vi "Simulador 22_03.vi"() -> ()   [LabVIEW 2014]
uses:
  <vilib>/imath/engines/lvmath2/RunTimeEngine/Managers/WorkSpace/UID Generator.vi
  <vilib>/imath/engines/lvmath2/RunTimeEngine/RunTimeType/NIMS_RunTimeType_From StrictType (excl LVString).vi
  <instcachedir>/0/NIMS_RunTimeType_From StrictType (excl LVString)_15A5391EEA9C4AACB9955AC755B83D29.lvgen/NIMS_RunTimeType_From StrictType (excl LVString)_15A5391EEA9C4AACB9955AC755B83D29_000.vi
  <vilib>/imath/engines/lvmath2/RunTimeEngine/LocalVariableDefStatement/MC_LocalVariableDefStatement_Display.vi
  <vilib>/imath/engines/lvmath2/RunTimeEngine/ArithmeticOperatorToken/NIMS_ArithmeticOperator_power(S).vi
  <instcachedir>/0/NIMS_ArithmeticOperator_power(S)_CAFE680B12A64A3A8F5E28A20C679B7D.lvgen/NIMS_ArithmeticOperator_power(S)_CAFE680B12A64A3A8F5E28A20C679B7D_010.vi
  <vilib>/imathl/engines/lvmath/Functions/Error Handling/Create Error.vi
  <vilib>/imath/engines/lvmath2/RunTimeEngine/Managers/SymbolTable/Clear UID.vi
  <vilib>/imath/engines/lvmath2/RunTimeEngine/NodeEndStatement/NIMS_NodeEndStatement_Output.vi
  <instcachedir>/0/NIMS_NodeEndStatement_Output_53EC0D466D134D7ABD903AC30B43404B.lvgen/NIMS_NodeEndStatement_Output_53EC0D466D134D7ABD903AC30B43404B_010.vi
  <instcachedir>/0/NIMS_NodeEndStatement_Output_53EC0D466D134D7ABD903AC30B43404B.lvgen/NIMS_NodeEndStatement_Output_53EC0D466D134D7ABD903AC30B43404B_001.vi
  <vilib>/imath/engines/lvmath2/RunTimeEngine/ErrorHandling/NIMS_Finalize Error.vi
  <vilib>/imath/engines/lvmath2/RunTimeEngine/Managers/SymbolTable/NIMS_WorkSpace.lvlib
panel:
  in  "h":cdb
  in  "milliseconds to wait":u32
  out "y":dbl
  in  "Present (s)":dbl
  out "Waveform Chart":dbl(graph)
  in  "stop":bool
  out "Tank":dbl(slide) scale=0.0..30.0
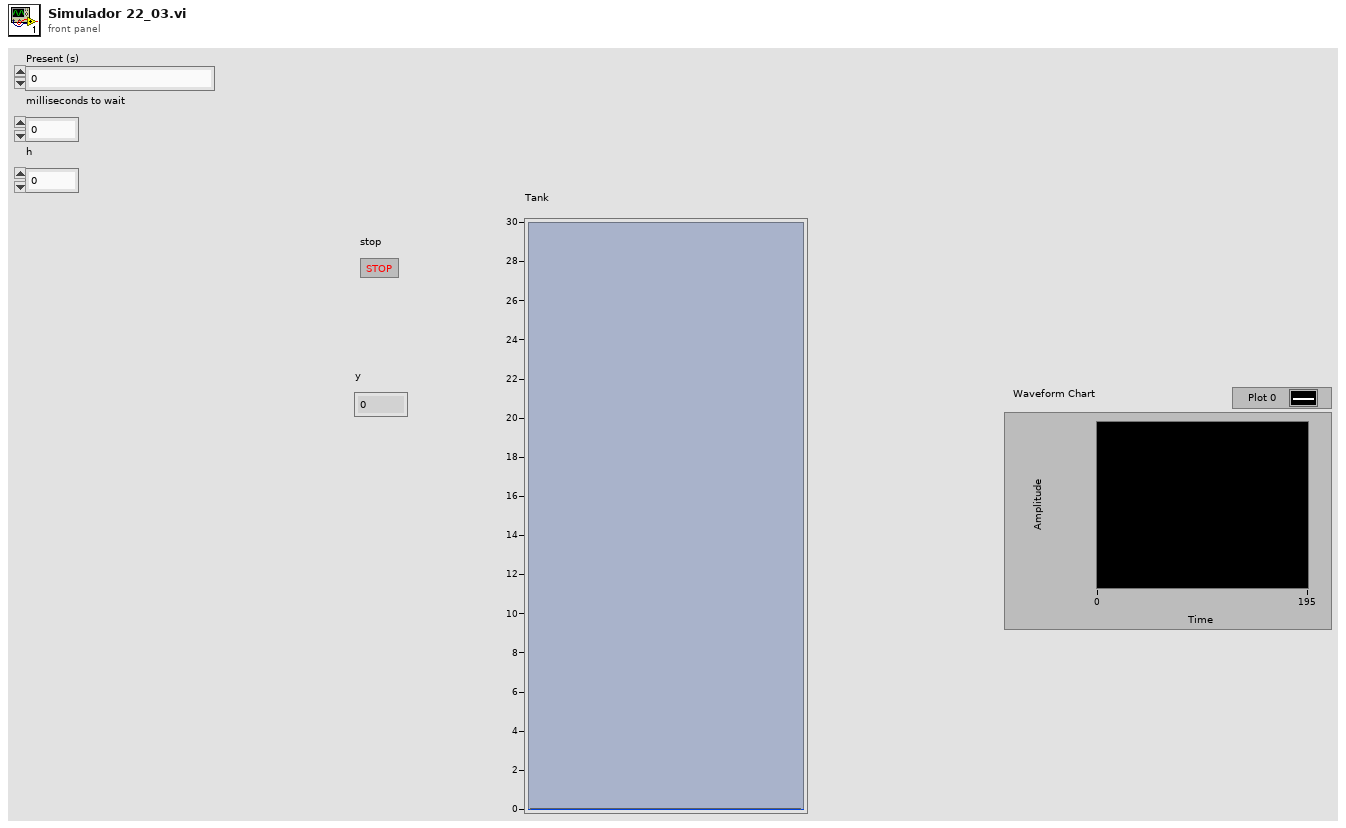
[diagram p1: front panel]
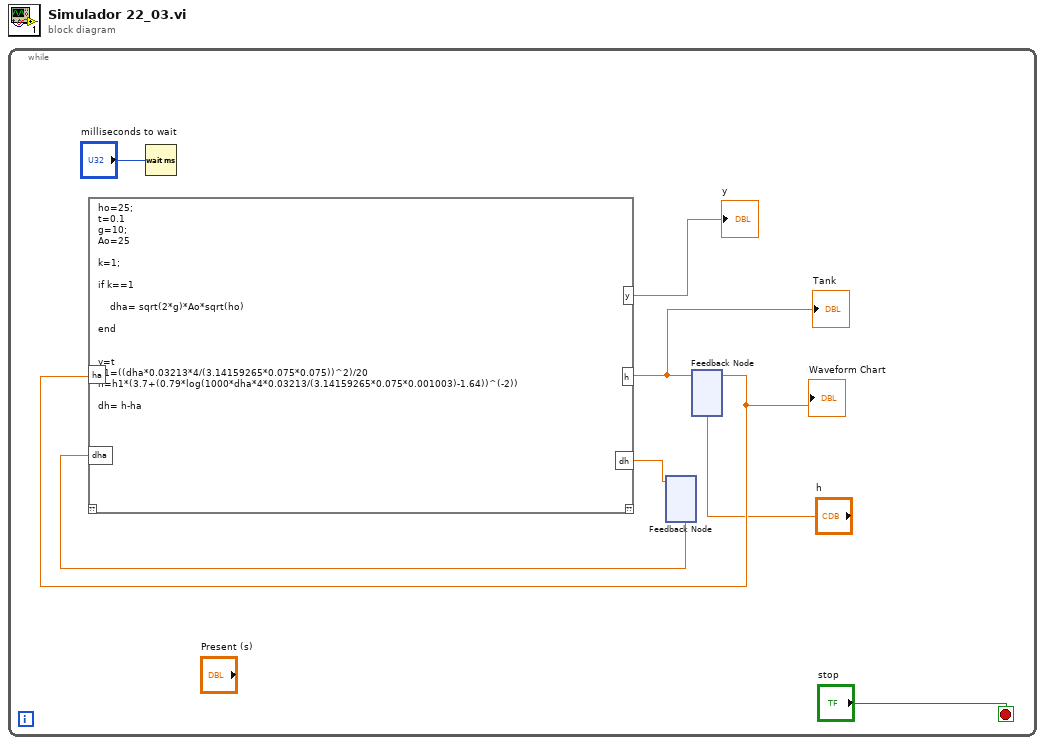
[diagram p0: block diagram]
diagram:
  n1 = while {
    stop <- "stop" stop-if-true
    n2 = Wait (ms)(milliseconds to wait="milliseconds to wait") -> ()  [unwired: 1 out]
    n3 = feedback #1() -> (w1:cdb)  [unwired: 1 in]
    n4 = feedback #2("h") -> (w8:cdb)
    "Tank" <- w8
    n5 = mathscript code="ho=25;\nt=0.1\ng=10;\nAo=25\n\nk=1;\n\nif k==1\n\n    dha= sqrt(2*g)*Ao*sqrt(ho)\n\nend\n\n\ny=t\nh1=((dha*0.03213*4/(3.14159265*0.075*0.075))^2)/20\nh=h1*(3.7+(0.79*log(1000*dha*4*0.03213/(3.14159265*0.075*0.001003)-1.64))^(-2))\n\ndh= h-ha"("ha"=w8, "dha"=w1) -> ("h"=w6:cdb, "y"=→"y":dbl, "dh"=w2:cdb)  [unwired: 1 in, 1 out]
    "Waveform Chart" <- w6
    n6 = feedback-in #1(w2) -> ()
    n7 = feedback-in #2(w6) -> ()
  }
